vi "NI VeriStand - Get Target Type.vi"(8 "error in (no error)":errorcluster, 11 "Node U64 ID":T2 format="%.0x") -> (0 "error out":errorcluster, 3 "Operating System":T1)   [LabVIEW 2026, in "Custom Devices Storage.lvlib"]
uses:
  Custom Devices Storage.lvlib
  <vilib>/NI VeriStand/Custom Device API/Custom Device Item Ref.ctl
  <vilib>/NI VeriStand/Custom Device API/Custom Device Target Type.ctl
  C:/Users/Administrator/Desktop/Jatin/All DNC DLLs/NationalInstruments.VeriStand.SystemDefinitionAPI.dll
  Jatin/All DNC DLLs/NationalInstruments.VeriStand.SystemDefinitionAPI.dll
  C:/Users/Administrator/Desktop/Jatin/All DNC DLLs/NationalInstruments.VeriStand.SystemStorage.dll
  Jatin/All DNC DLLs/NationalInstruments.VeriStand.SystemStorage.dll
  <vilib>/NI VeriStand/Custom Device API/Custom Device API.lvlib
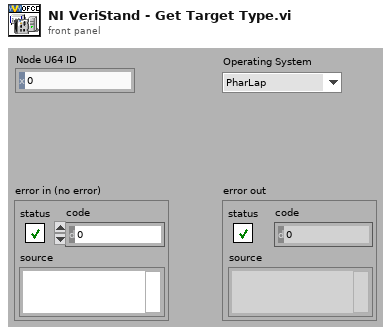
[diagram p1: front panel]
types:
  T1 = typedef "Custom Device API.lvlib/Custom Device Target Type.ctl" = enum16{"PharLap", "VxWorks", "Windows", "Linux_32_ARM", "Linux_x64"}
  T2 = typedef "Custom Device API.lvlib/Custom Device Item Ref.ctl" = u64
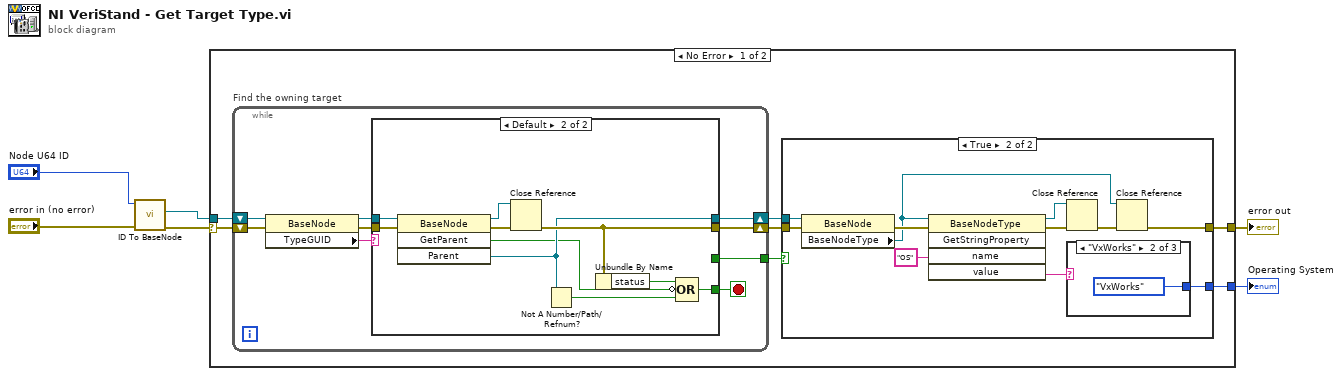
[diagram p0: block diagram]
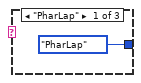
[diagram p3: hidden frame]
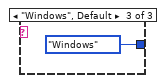
[diagram p4: hidden frame]
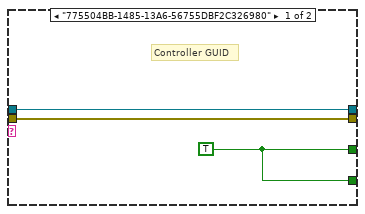
[diagram p5: hidden frame]
diagram:
  n1 = call "ID To BaseNode.vi"("error in (no error)"="error in (no error)", "ID in"="Node U64 ID") -> ("error out"=w4:errorcluster, "NationalInstruments.VeriStand.SystemDefinitionAPI.BaseNode"=w3:refnum<k39>)  [unwired: 7 in, 1 out]
  n2 = case shown="No Error" w4 {
    selector: w4 -> [w13 w51]
    tunnel: w3 -> [w12 _]
    tunnel: [w7 w51] -> w2
    tunnel: [w8 _] -> w1
    frame No Error {
      n3 = while "Find the owning target" {
        shift-right: [w36] -> w11
        shift-left: w13 -> [w33]
        shift-right: [w35] -> w9
        shift-left: w12 -> [w32]
        tunnel: [w34] -> w10
        stop <- w37 stop-if-true
        n4 = property class="BaseNode"(reference=w32, error in=w33) -> (reference out=w29:refnum<k39>, error out=w30:errorcluster, "TypeGUID"=w31:string)
        n5 = case shown="Default" w31 {
          tunnel: w30 -> [w39 w47]
          tunnel: w29 -> [w40 w46]
          tunnel: [w38 w48] -> w37
          tunnel: [w39 w50] -> w36
          tunnel: [w40 w45] -> w35
          tunnel: [w38 _] -> w34
          frame "775504BB-1485-13A6-56755DBF2C326980" {
            w38 = TRUE
            # "Controller GUID"
          }
          frame Default {
            n6 = invoke class="BaseNode" method="GetParent"(reference=w46, error in=w47) -> (reference out=w43:refnum<k39>, error out=w44:errorcluster, "GetParent"=w41:bool, "Parent"=w45:refnum<k39>)  [unwired: 2 in]
            n7 = Close Reference(reference=w43, error in (no error)=w44) -> (error out=w50:errorcluster)
            n8 = Not A Number/Path/Refnum?(number/path/refnum=w45) -> (NaN/Path/Refnum?=w42:bool)
            n9 = Unbundle By Name(w50) -> ("status"=w49:bool)
            n10 = Compound Arithmetic op=OR(w49, invert w41, w42) -> (w48:bool)
          }
        }
      }
      n11 = case shown="True" w10 {
        tunnel: w11 -> [w14 w25]
        tunnel: w9 -> [_ w23]
        tunnel: [_ w20] -> w8
        tunnel: [w14 w15] -> w7
        frame False {
        }
        frame True {
          n12 = property class="BaseNode"(reference=w23, error in=w25) -> (error out=w24:errorcluster, "BaseNodeType"=w16:refnum<k39>)  [unwired: 1 out]
          n13 = invoke class="BaseNodeType" method="GetStringProperty"(reference=w16, error in=w24, "name"="OS") -> (reference out=w18:refnum<k39>, error out=w19:errorcluster, "value"=w21:string)  [unwired: 2 in, 2 out]
          n14 = Close Reference(reference=w18, error in (no error)=w19) -> (error out=w17:errorcluster)
          n15 = case shown="\"VxWorks\"" w21 {
            tunnel: [Custom_Device_Target_Type."PharLap" ("Operating System") Custom_Device_Target_Type."VxWorks" ("Operating System") Custom_Device_Target_Type."Windows" ("Operating System")] -> w20
            frame "PharLap" {
            }
            frame "VxWorks" {
            }
            frame "Windows", Default {
            }
          }
          n16 = Close Reference(reference=w16, error in (no error)=w17) -> (error out=w15:errorcluster)
        }
      }
    }
    frame Error {
    }
  }
  "error out" <- w2
  "Operating System" <- w1
